vi "MAT Read Matrix Header.vi"(8 "Error In":errorcluster, 11 "Ref Num":refnum<file>) -> (0 "error out":errorcluster, 1 "offset":i32, 2 "Matrix Name":string, 3 "Dup Ref Num":refnum<file>, 4 "Real/Complex (0 - Real)":u32, 5 "Matrix Size (rows x cols)":i32[](array[numeric]), 6 "Rep. Code":u32)   [LabVIEW 2020, in "varilib.lvlib"]
uses:
  varilib.lvlib
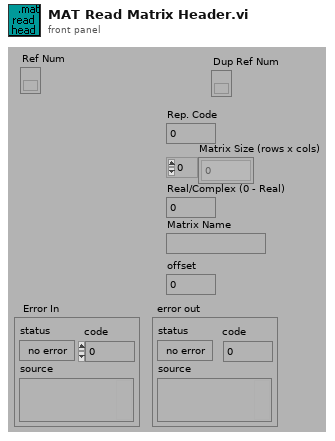
[diagram p1: front panel]
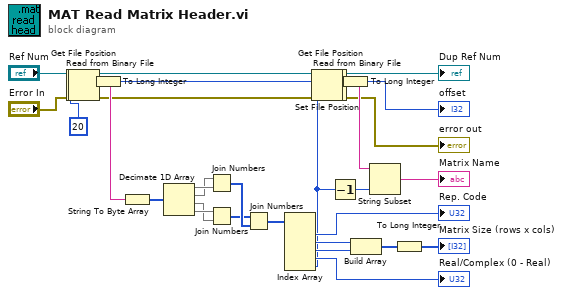
[diagram p0: block diagram]
diagram:
  n1 = Read from Binary File(8:"Error In", 10:20 ("count"), 11:"Ref Num") -> (0:w2:errorcluster, 2:w36:string, 3:w3:refnum<file>)  [unwired: 3 in, 1 out]
  n2 = Get File Position(4:w2, 7:w3) -> (0:w23:errorcluster, 2:w1:i64, 3:w22:refnum<file>)
  n3 = To Long Integer(number=w1) -> (32bit integer=w9:i32)
  n4 = String To Byte Array(string=w36) -> (unsigned byte array=w34:u8[])
  n5 = Decimate 1D Array(w34) -> (w33:u8[], w32:u8[], w11:u8[], w12:u8[])
  n6 = Join Numbers(hi=w32, lo=w33) -> ((hi.lo)=w31:u16[])
  n7 = Join Numbers(hi=w12, lo=w11) -> ((hi.lo)=w10:u16[])
  n8 = Join Numbers(hi=w10, lo=w31) -> ((hi.lo)=w30:u32[])
  n9 = Index Array(array=w30) -> (element #1=→"Rep. Code":u32, element #2=w28:u32, element #3=w27:u32, element #4=→"Real/Complex (0 - Real)":u32, element #5=w21:u32)  [unwired: 5 in]
  n10 = Set File Position(offset (in bytes) (0)=w9, refnum=w22, error in=w23) -> (refnum out=w8:refnum<file>, error out=w7:errorcluster)  [unwired: 1 in]
  n11 = Read from Binary File(8:w7, 10:w21, 11:w8) -> (0:w5:errorcluster, 2:w19:string, 3:w6:refnum<file>)  [unwired: 3 in, 1 out]
  n12 = Get File Position(4:w5, 7:w6) -> (0:→"error out":errorcluster, 2:w4:i64, 3:→"Dup Ref Num":refnum<file>)
  n13 = Decrement(x=w21) -> (x-1=w20:u32)
  n14 = To Long Integer(number=w4) -> (32bit integer=→"offset":i32)
  n15 = Build Array(w28, w27) -> (w26:u32[])
  n16 = String Subset(string=w19, length (rest)=w20) -> (substring=→"Matrix Name":string)  [unwired: 1 in]
  n17 = To Long Integer(number=w26) -> (32bit integer=→"Matrix Size (rows x cols)":i32[])
